vi "Teleop Intake Control.vi"(0 "Driver Button Cluster":T2, 1 "Manipulator Button Cluster":T2, 2 "Manipulator Axes":T1, 3 "Driver Axes":T1) -> ()   [LabVIEW 2015]
uses:
  Common Code/Gamepads/Button Cluster.ctl
  Common Code/Gamepads/Axes Cluster.ctl
  Common Code/Intake Commands.ctl
  Common Code/Change Detect.vi
  Common Code/Change Detect Boolean.vi
  Robot Global Data.vi
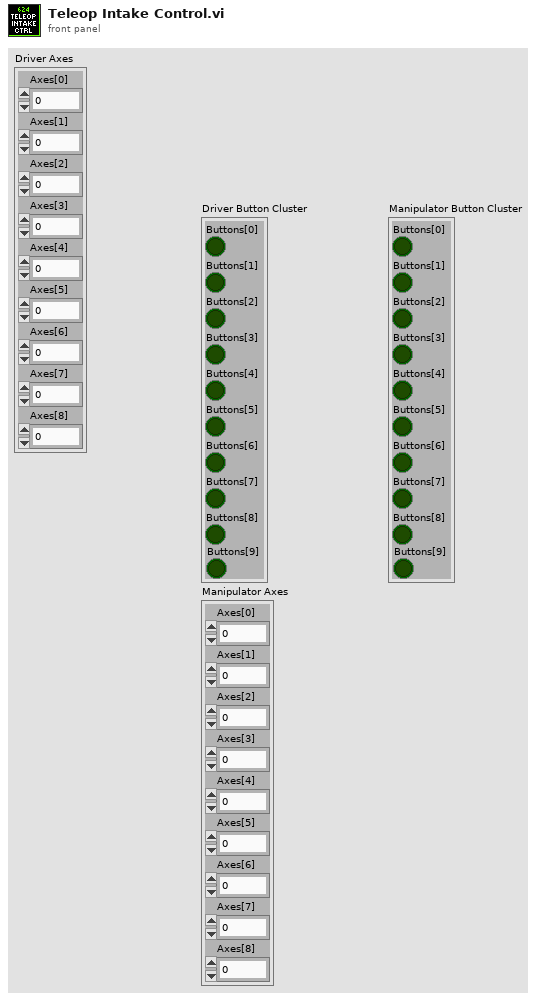
[diagram p1: front panel]
types:
  T1 = typedef "Axes Cluster.ctl" = cluster{"Axes[0]":dbl, "Axes[1]":dbl, "Axes[2]":dbl, "Axes[3]":dbl, "Axes[4]":dbl, "Axes[5]":dbl, "Axes[6]":dbl, "Axes[7]":dbl, "Axes[8]":dbl}
  T2 = typedef "Button Cluster.ctl" = cluster{"Buttons[0]":bool, "Buttons[1]":bool, "Buttons[2]":bool, "Buttons[3]":bool, "Buttons[4]":bool, "Buttons[5]":bool, "Buttons[6]":bool, "Buttons[7]":bool, "Buttons[8]":bool, "Buttons[9]":bool}
  T3 = typedef "Intake Commands.ctl" = enum16{"Unload", "Load", "Pull up", "Drop low", "Idle", "Lift Half"}
  T4 = enum16{"0", "1", "2", "3", "4", "5", "6", "7", "8", "9", "A", "B", "C", "D", "E", "F", "G", "H", "I", "J", "K", "L", "M", "N", "O", "P", "Q", "R", "S", "T", "U", "V", "W", "X", "Y", "Z", "F1", "F2", "F3", "F4", "F5", "F6", "F7", "F8", "F9", "F10", "F11", "F12", "F13", "F14", "F15", "ADD", "BACK", "BACKSLASH", "CAPITAL", "COMMA", "DECIMAL", "DELETE", "DIVIDE", "DOWN", "END", "EQUALS", "ESCAPE", "GRAVE (`)", "HOME", "INSERT", "LBRACKET", "LCONTROL", "LEFT", "L ALT", "LSHIFT", "LWIN", "MINUS", "MULTIPLY", "NEXT", "NUMLOCK", "NUMPAD_0", "NUMPAD_1", "NUMPAD_2", "NUMPAD_3", "NUMPAD_4", "NUMPAD_5", "NUMPAD_6", "NUMPAD_7", "NUMPAD_8", "NUMPAD_9", "PAUSE", "PERIOD", "PRIOR (PG UP)", "RBRACKET", "RCONTROL", "RETURN", "RIGHT", "R ALT", "RSHIFT", "RWIN", "SCROLL", "SEMICOLON", "SLASH", "SPACE", "SUBTRACT", "TAB", "UP", "ENTER (num pad)", "' (quote)"}
  T5 = typedef "Intake Commands Cluster.ctl" = cluster{"Intake Commands":T3, "Intake Mode":T6, "Override IR":bool}
  T6 = typedef "Intake Mode.ctl" = enum16{"Safe", "Auto", "Manual"}
  T7 = typedef "Manual Intake Commands.ctl" = cluster{"Intake":bool, "Eject":bool, "Arm Angle":dbl, "Intake Override Speed":dbl, "Arm Override Speed":dbl, "Arm Speed":dbl, "Override Intake":bool, "Override Eject":bool, "Eject Override Speed":dbl, "Arm":bool, "Override Arm":bool}
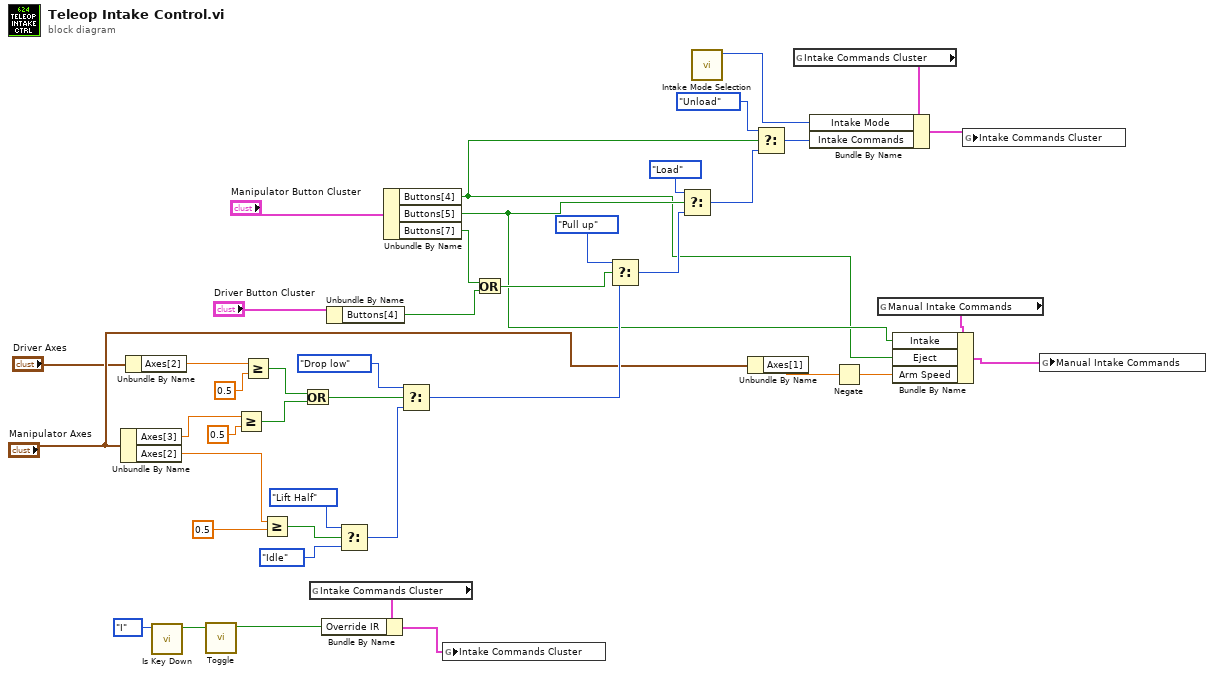
[diagram p0: block diagram]
diagram:
  n1 = Unbundle By Name("Manipulator Axes") -> ("Axes[3]"=w34:dbl, "Axes[2]"=w29:dbl)
  n2 = Unbundle By Name("Driver Axes") -> ("Axes[2]"=w15:dbl)
  n3 = call "Is Key Down.vi"("Key"=T4."I") -> ("Key Down?"=w7:bool)  [unwired: 10 in]
  n4 = call "Toggle.vi"("In"=w7) -> ("Toggled"=w8:bool)  [unwired: 10 in]
  n5 = Greater Or Equal?(x=w34, y=0.5) -> (x >= y?=w13:bool)
  n6 = Greater Or Equal?(x=w15, y=0.5) -> (x >= y?=w14:bool)
  n7 = Greater Or Equal?(x=w29, y=0.5) -> (x >= y?=w26:bool)
  n8 = Or(x=w14, y=w13) -> (x .or. y?=w12:bool)
  n9 = global read "Robot Global Data.vi" "Intake Commands Cluster"() -> (w5:T5)
  n10 = Bundle By Name(cluster=w5, "Override IR"=w8) -> (w9:T5)
  n11 = Unbundle By Name("Driver Button Cluster") -> ("Buttons[4]"=w37:bool)
  n12 = Select(t=Intake_Commands."Lift Half" ("f"), s=w26, f=Intake_Commands."Idle") -> (s? t:f=w27:T3)
  n13 = Unbundle By Name("Manipulator Button Cluster") -> ("Buttons[4]"=w11:bool, "Buttons[5]"=w18:bool, "Buttons[7]"=w10:bool)
  n14 = Select(t=Intake_Commands."Drop low" ("Intake Commands"), s=w12, f=w27) -> (s? t:f=w31:T3)
  n15 = global write "Robot Global Data.vi" "Intake Commands Cluster"(w9) -> ()
  n16 = Or(x=w10, y=w37) -> (x .or. y?=w22:bool)
  n17 = Select(t=Intake_Commands."Pull up" ("Intake Commands"), s=w22, f=w31) -> (s? t:f=w39:T3)
  n18 = Select(t=Intake_Commands."Load" ("Intake Commands"), s=w18, f=w39) -> (s? t:f=w24:T3)
  n19 = call "Intake Mode Selection.vi"() -> ("Mode"=w19:T6)  [unwired: 11 in]
  n20 = Unbundle By Name("Manipulator Axes") -> ("Axes[1]"=w20:dbl)
  n21 = Select(t=Intake_Commands."Unload" ("Intake Commands"), s=w11, f=w24) -> (s? t:f=w25:T3)
  n22 = global read "Robot Global Data.vi" "Intake Commands Cluster"() -> (w36:T5)
  n23 = Bundle By Name(cluster=w36, "Intake Mode"=w19, "Intake Commands"=w25) -> (w35:T5)
  n24 = Negate(x=w20) -> (-x=w3:dbl)
  n25 = global read "Robot Global Data.vi" "Manual Intake Commands"() -> (w2:T7)
  n26 = Bundle By Name(cluster=w2, "Intake"=w18, "Eject"=w11, "Arm Speed"=w3) -> (w4:T7)
  n27 = global write "Robot Global Data.vi" "Intake Commands Cluster"(w35) -> ()
  n28 = global write "Robot Global Data.vi" "Manual Intake Commands"(w4) -> ()
